vi "AutoRunFromPlayback.vi"(8 "error in (no error)":errorcluster, 10 "ControlValueUpdates[] in":T1[](array[typedef]), 11 "UI_Interaction_Manager in":refnum<class "UI_Interaction_Manager.lvclass">) -> (0 "error out":errorcluster, 3 "UI_Interaction_Manager out":refnum<class "UI_Interaction_Manager.lvclass">)   [LabVIEW 2011, in "UI_Interaction_Manager.lvclass"]
uses:
  UI_Interaction_Manager.lvclass
  TypeDefs/ControlValueUpdate.ctl
  UI_Interaction_Manager.lvclass/UI_Interaction_Manager.ctl
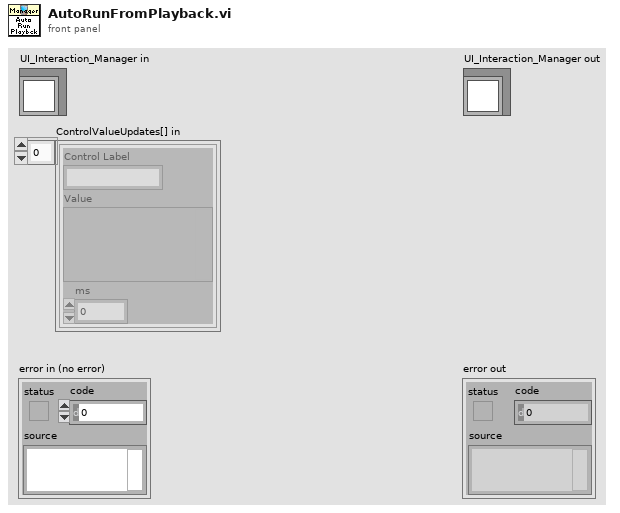
[diagram p1: front panel]
types:
  T1 = typedef "UI_Interaction_Manager.lvclass/ControlValueUpdate.ctl" = cluster{"Control Label":string, "Value":variant, "ms":u32}
  T2 = enum8{"Enabled", "Disabled", "Disabled and Grayed Out"}
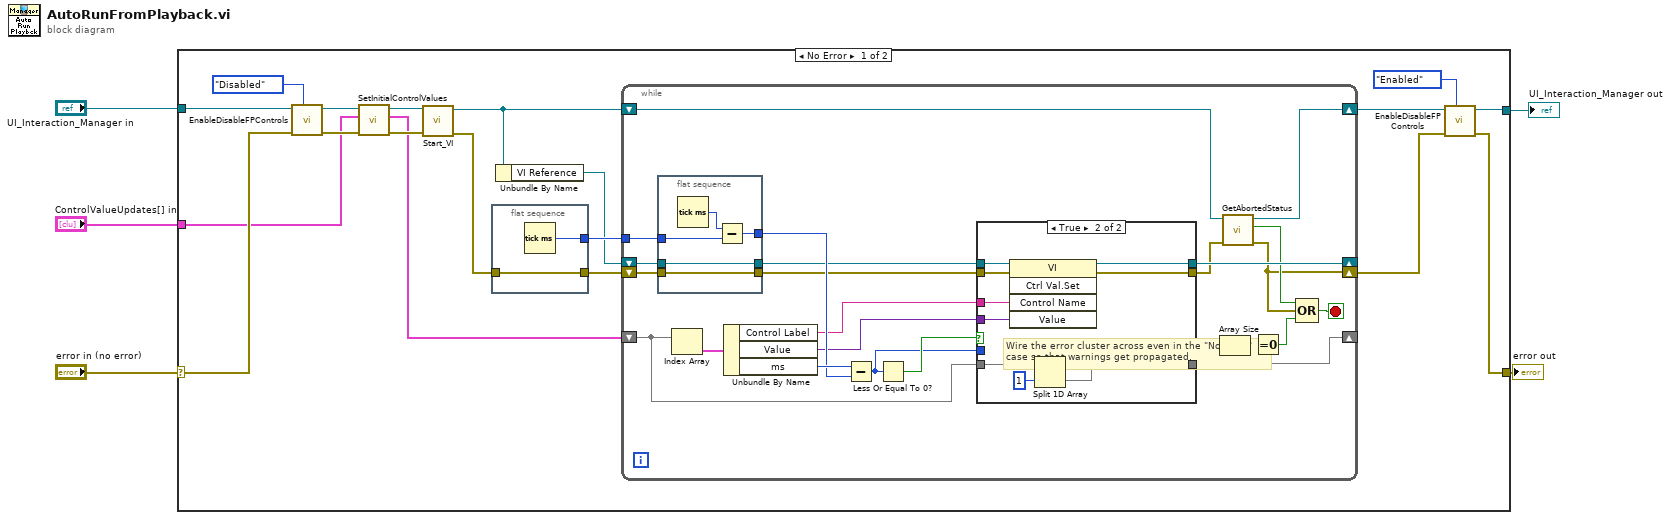
[diagram p0: block diagram]
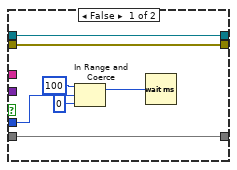
[diagram p2: hidden frame]
diagram:
  n1 = case shown="No Error" "error in (no error)" {
    selector: "error in (no error)" -> [w24 w72]
    tunnel: [w21 w72] -> w4
    tunnel: [w22 w71] -> w2
    tunnel: "UI_Interaction_Manager in" -> [w11 w71]
    tunnel: "ControlValueUpdates[] in" -> [w17 _]
    frame No Error {
      # "Wire the error cluster across even in the \"No Error\"\ncase so that warnings get propagated."
      n2 = call "EnableDisableFPControls.vi"("Enable/Disable?"=T2."Disabled", "error in (no error)"=w24, "UI_Interaction_Manager in"=w11) -> ("error out"=w18:errorcluster, "UI_Interaction_Manager out"=w19:refnum<class "UI_Interaction_Manager.lvclass">)  [unwired: 7 in]
      n3 = call "SetInitialControlValues.vi"("error in (no error)"=w18, "ControlValueUpdates[] in"=w17, "UI_Interaction_Manager in"=w19) -> ("error out"=w16:errorcluster, "ControlValueUpdates[] out"=w9:T1[], "UI_Interaction_Manager out"=w15:refnum<class "UI_Interaction_Manager.lvclass">)  [unwired: 6 in]
      n4 = call "Start_VI.vi"("error in (no error)"=w16, "UI_Interaction_Manager in"=w15) -> ("error out"=w12:errorcluster, "UI_Interaction_Manager out"=w8:refnum<class "UI_Interaction_Manager.lvclass">)  [unwired: 8 in]
      n5 = flat-sequence {
        tunnel: [w70] -> w14
        tunnel: [w69] -> w13
        tunnel: w12 -> [w69]
        frame #0 {
          n6 = Tick Count (ms)() -> (millisecond timer value=w70:u32)
        }
      }
      n7 = Unbundle By Name(w8) -> ("VI Reference"=w10:refnum<vi>)
      n8 = while {
        shift-right: [w47] -> _
        shift-left: w10 -> [w46]
        tunnel: w14 -> [w45]
        shift-right: [w35] -> _
        shift-left: w9 -> [w40]
        shift-right: [w25] -> w6
        shift-left: w13 -> [w32]
        shift-right: [w30] -> w7
        shift-left: w8 -> [w31]
        stop <- w28 stop-if-true
        n9 = flat-sequence {
          tunnel: w46 -> [w50]
          tunnel: w45 -> [w51]
          tunnel: [w50] -> w37
          tunnel: [w49] -> w42
          tunnel: [w48] -> w33
          tunnel: w32 -> [w48]
          frame #0 {
            n10 = Tick Count (ms)() -> (millisecond timer value=w52:u32)
            n11 = Subtract(x=w52, y=w51) -> (x-y=w49:u32)
          }
        }
        n12 = Index Array(array=w40) -> (element=w44:T1)  [unwired: 1 in]
        n13 = Unbundle By Name(w44) -> ("Control Label"=w39:string, "Value"=w38:variant, "ms"=w43:u32)
        n14 = Subtract(x=w43, y=w42) -> (x-y=w36:u32)
        n15 = Less Or Equal To 0?(x=w36) -> (x <= 0?=w41:bool)
        n16 = case shown="True" w41 {
          tunnel: w37 -> [w58 w68]
          tunnel: w38 -> [_ w67]
          tunnel: w40 -> [w59 w66]
          tunnel: [w59 w64] -> w35
          tunnel: [w58 w63] -> w47
          tunnel: w39 -> [_ w62]
          tunnel: w36 -> [w57 _]
          tunnel: w33 -> [w53 w61]
          tunnel: [w53 w60] -> w29
          frame False {
            n17 = In Range and Coerce(upper limit=u32 100, x=w57, lower limit=u32 0) -> (coerced(x)=w54:u32)  [unwired: 1 out]
            n18 = Wait (ms)(milliseconds to wait=w54) -> ()  [unwired: 1 out]
          }
          frame True {
            n19 = invoke class="VI" method="Ctrl Val.Set"(reference=w68, error in=w61, "Control Name"=w62, "Value"=w67) -> (reference out=w63:refnum<vi>, error out=w60:errorcluster)  [unwired: 1 in, 3 out]
            n20 = Split 1D Array(array=w66, index=1) -> (second subarray=w64:T1[])  [unwired: 1 out]
          }
        }
        n21 = Array Size(array=w35) -> (size(s)=w34:i32)
        n22 = call "GetAbortedStatus.vi"("error in (no error)"=w29, "UI_Interaction_Manager in"=w31) -> ("error out"=w25:errorcluster, "Aborted?"=w26:bool, "UI_Interaction_Manager out"=w30:refnum<class "UI_Interaction_Manager.lvclass">)  [unwired: 7 in]
        n23 = Equal To 0?(x=w34) -> (x = 0?=w27:bool)
        n24 = Compound Arithmetic op=OR(w26, w25, w27) -> (w28:bool)
      }
      n25 = call "EnableDisableFPControls.vi"("Enable/Disable?"=T2."Enabled", "error in (no error)"=w6, "UI_Interaction_Manager in"=w7) -> ("error out"=w21:errorcluster, "UI_Interaction_Manager out"=w22:refnum<class "UI_Interaction_Manager.lvclass">)  [unwired: 7 in]
    }
    frame Error {
    }
  }
  "error out" <- w4
  "UI_Interaction_Manager out" <- w2
